vi "Robot Global Data.vi"() -> ()   [LabVIEW 2018]
doc: "This global VI can contain as many global variables as you need. Place a control on the panel, give it a good name. To read or write to it from a VI, drag the icon to the diagram of that VI. You can also drag from the project. Click on the node to change which global you access. You shouldn't have multiple locations writing to a global or it will cause a race-condition."
uses:
  <vilib>/Rock Robotics/WPI/DriverStation/WPI_DriverStationRobotMode2.ctl
panel:
  in  "Right Side Auto":bool
  in  "Auto End Override":bool
  out "Has Visited Auto?":bool
  in  "Auto to Run":string="Fun Rocket Close"
  out "Autonomous":bool=TRUE
  out "Trying to Drive":bool
  in  "Limelight Pipeline":dbl
  in  "Limelight Cam Mode":dbl
  in  "Limelight Led Mode":dbl
  in  "Limelight Data":T1={"offsetAngle H"=0.0, "offsetAngle V"=0.0, "area"=0.0, "skew"=0.0, "validTarget"=0.0, "latency"=8.333280563354492}
  in  "Robot Mode":T2=enum."Teleop Disabled"
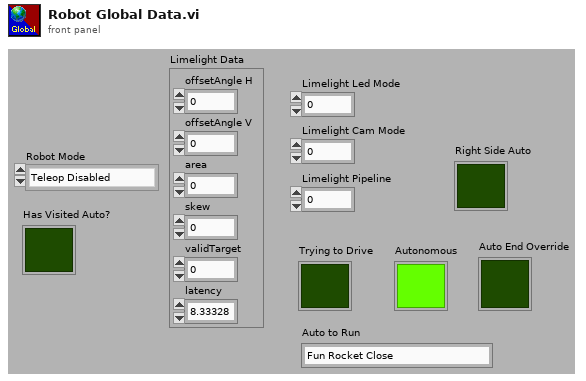
[diagram p1: front panel]
types:
  T1 = cluster{"offsetAngle H":dbl, "offsetAngle V":dbl, "area":dbl, "skew":dbl, "validTarget":dbl, "latency":dbl}
  T2 = typedef "WPI_DriverStationRobotMode2.ctl" = enum16{"Autonomous Disabled", "Autonomous Enabled", "Teleop Disabled", "Teleop Enabled", "Disconnected", "Finish", "Test Disabled", "Test Enabled", "Emergency Stopped"}
diagram:
